vi "Active Pumps.vi"(5 "Action (F:Read)":bool, 6 "Remove Pump (F)":bool, 7 "Pump ID (0:A)":T1, 8 "error in (no error)":errorcluster, 9 "Value in":dbl, 10 "Parameter":T2, 11 "VISA resource in":refnum<visa-resource-name>) -> (0 "error out":errorcluster, 1 "Value out":dbl, 2 "Found":bool, 3 "VISA resource out":refnum<visa-resource-name>)   [LabVIEW 2020, in "Global FIA milliGAT.lvlib"]
uses:
  <instrlib>/RxnRover/Global FIA milliGAT 3.14/Global FIA milliGAT.lvlib
  <instrlib>/RxnRover/Global FIA milliGAT 3.14/Private/Pump Parameter.ctl
  <instrlib>/RxnRover/Global FIA milliGAT 3.14/Public/Utility/Pump Address.ctl
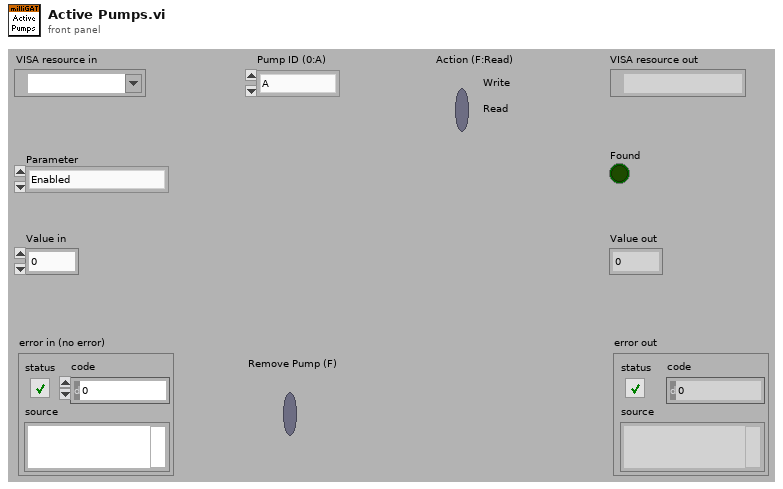
[diagram p1: front panel]
types:
  T1 = typedef "Global FIA milliGAT.lvlib/Pump Address.ctl" = enum16{"A", "B", "C", "D", "E", "F", "G", "H", "I", "J", "K", "L", "M", "N", "O", "P", "Q", "R", "S", "T", "U", "V", "W", "X", "Y", "Z", "a", "b", "c", "d", "e", "f", "g", "h", "i", "j", "k", "l", "m", "n", "o", "p", "q", "r", "s", "t", "u", "v", "w", "x", "y", "z", "0", "1", "2", "3", "4", "5", "6", "7", "8", "9"}
  T2 = typedef "Global FIA milliGAT.lvlib/Pump Parameter.ctl" = enum16{"Enabled", "EU", "EU Calibration Factor", "Fixed Asp or Disp", "Starting Position", "Starting Flow", "Peak Flow", "Flow Acceleration", "Flow Deceleration", "Session Volume", "Max Pressure", "Backlash (usteps)", "BL Calibration Factor", "BL Correction Enabled", "Min Flow", "Max Flow", "Min Acceleration", "Max Acceleration", "Service Volume", "Life Volume"}
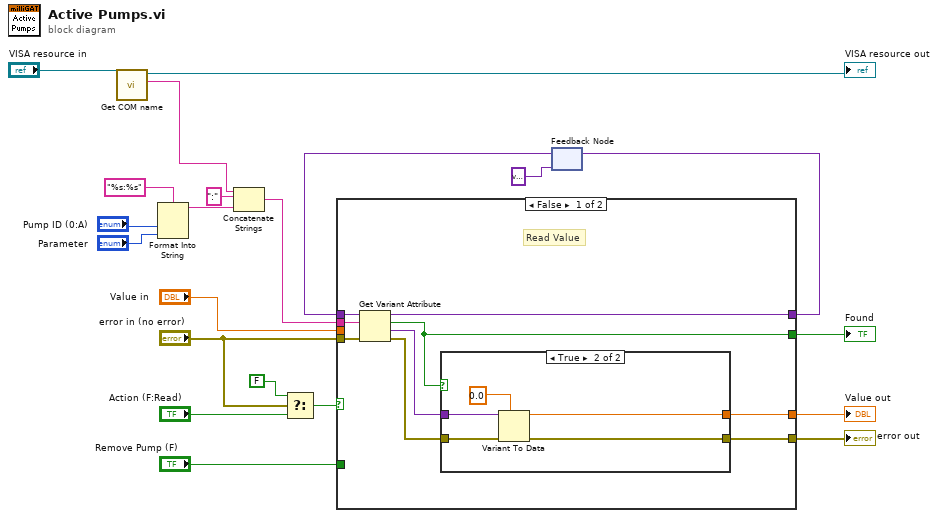
[diagram p0: block diagram]
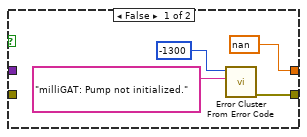
[diagram p2: hidden frame]
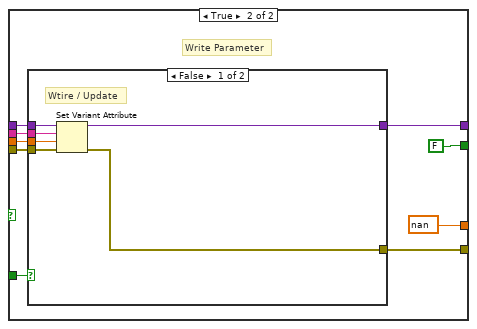
[diagram p3: hidden frame]
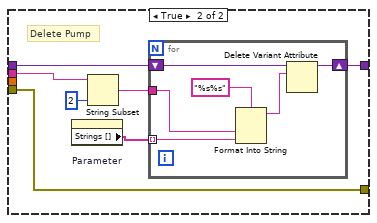
[diagram p4: hidden frame]
diagram:
  n1 = call <instrlib>:"Get COM name.vi"("VISA resource in"="VISA resource in") -> ("COM name"=w1:string, "VISA resource out"=→"VISA resource out":refnum<visa-resource-name>)  [unwired: 8 in, 1 out]
  n2 = Format Into String(format string="%s:%s", "Pump ID (0:A)", "Parameter") -> (resulting string=w5:string)  [unwired: 2 in, 1 out]
  n3 = Concatenate Strings(w1, ":", w5) -> (w4:string)
  n4 = Select(t=FALSE, s="error in (no error)", f="Action (F:Read)") -> (s? t:f=w11:bool)
  n5 = feedback #1(variant) -> (w21:variant)
  n6 = case shown="False" w11 {
    tunnel: w21 -> [w30 w48]
    tunnel: [w29 w47] -> w20
    tunnel: w4 -> [w28 w46]
    tunnel: "Value in" -> [_ w45]
    tunnel: [w23 FALSE] -> w15
    tunnel: [w25 w43] -> w9
    tunnel: [w24 nan ("Value out")] -> w14
    tunnel: "error in (no error)" -> [w22 w41]
    tunnel: "Remove Pump (F)" -> [_ w40]
    frame False {
      # "Read Value"
      n7 = Get Variant Attribute(Variant=w30, name=w28, error in=w22) -> (duplicate Variant=w29:variant, found=w23:bool, value=w27:variant, error out=w26:errorcluster)  [unwired: 1 in]
      n8 = case shown="True" w23 {
        tunnel: w27 -> [_ w39]
        tunnel: w26 -> [_ w38]
        tunnel: [w31 w36] -> w25
        tunnel: [nan ("Value out") w35] -> w24
        frame False {
          n9 = call <vilib>:"Error Cluster From Error Code.vi"("error message (\"\")"="milliGAT: Pump not initialized." ("error message (\"\")"), "error code (0)"=-1300) -> ("error out"=w31:errorcluster)  [unwired: 7 in]
        }
        frame True {
          n10 = Variant To Data(error in=w38, type=0.0 ("Value out"), Variant=w39) -> (data=w35:dbl, error out=w36:errorcluster)
        }
      }
    }
    frame True {
      # "Write Parameter"
      n11 = case shown="False" w40 {
        tunnel: w48 -> [w54 w59]
        tunnel: [w53 w61] -> w47
        tunnel: w46 -> [w52 w58]
        tunnel: w45 -> [w51 _]
        tunnel: [w50 w60] -> w43
        tunnel: w41 -> [w49 w60]
        frame False {
          # "Wtire / Update"
          n12 = Set Variant Attribute(Variant=w54, name=w52, value=w51, error in=w49) -> (Variant out=w53:variant, error out=w50:errorcluster)  [unwired: 1 out]
        }
        frame True {
          # "Delete Pump"
          n13 = property on="Parameter" class="Enum (strict)"() -> ("Strings []"=w55:string[])  [unwired: 2 in, 2 out]
          n14 = String Subset(string=w58, length (rest)=2 ("length (rest)")) -> (substring=w56:string)  [unwired: 1 in]
          n15 = for {
            shift-right: [w67] -> w61
            shift-left: w59 -> [w66]
            tunnel: w56 -> [w64]
            tunnel: w55 -> [w63] mode=indexing
            n16 = Format Into String(format string="%s%s", w64, w63) -> (resulting string=w62:string)  [unwired: 2 in, 1 out]
            n17 = Delete Variant Attribute(6:w62, 7:w66) -> (3:w67:variant)  [unwired: 1 in, 2 out]
          }
        }
      }
    }
  }
  "Value out" <- w14
  "error out" <- w9
  "Found" <- w15
  n18 = feedback-in #1(w20) -> ()
